vi "Initialize.vi"(8 "error in":errorcluster, 10 "shared resources":refnum<class "Shared Resources.lvclass">, 11 "Address Based Execution Unit Implementation in":refnum<class "Address Based Execution Unit.lvclass">) -> (0 "error out":errorcluster, 3 "Address Based Execution Unit Implementation out":refnum<class "Address Based Execution Unit.lvclass">)   [LabVIEW 2020, in "Ballard MIL-STD-1553 Engine.lvlib" / "Implementation.lvlib" / "Address Based Execution Unit.lvclass"]
uses:
  Address Based Execution Unit.lvclass
  Execution Unit/Execution Unit.lvclass
  Interfaces/Shared Resources/Shared Resources.lvclass
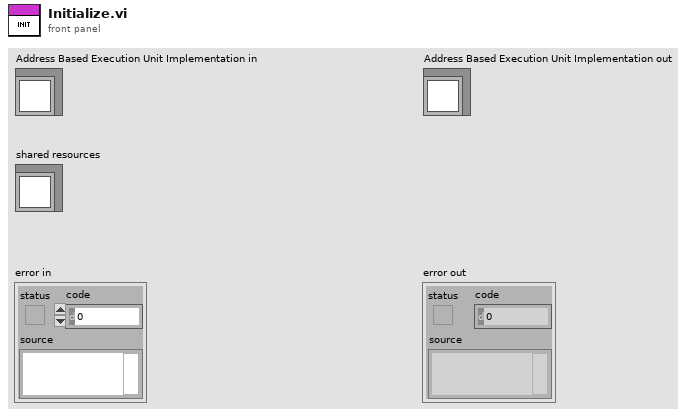
[diagram p1: front panel]
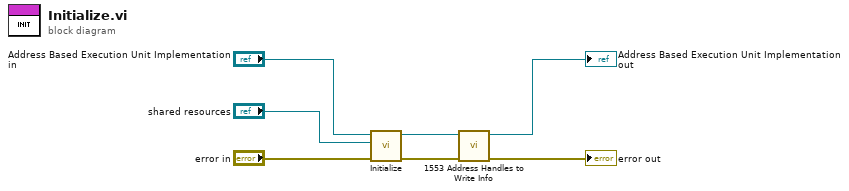
[diagram p0: block diagram]
diagram:
  n1 = call-parent "Initialize.vi"("error in"="error in", "shared resources"="shared resources", "Execution Unit Implementation in"="Address Based Execution Unit Implementation in") -> ("error out"=w4:errorcluster, "Execution Unit Implementation out"=w2:refnum<class "Address Based Execution Unit.lvclass">)  [unwired: 7 in]
  n2 = call "1553 Address Handles to Write Info.vi"("error in"=w4, "Address Based Execution Unit Implementation in"=w2) -> ("error out"=→"error out":errorcluster, "Address Based Execution Unit Implementation out"=→"Address Based Execution Unit Implementation out":refnum<class "Address Based Execution Unit.lvclass">)  [unwired: 8 in]
